vi "Add Dummy Grand Children.vi"(8 "error in (no error)":errorcluster, 9 "Folder Names":string[](array[string]), 10 "Parent Tag":string, 11 "Tree In":refnum<vi>) -> (0 "error out":errorcluster, 1 "Folder Names Dup":string[](array[string]), 2 "Parent Tag Dup":string, 3 "Tree Out":refnum<vi>)   [LabVIEW 2018, in "Tree Browser.lvlib"]
doc: "Adds a placeholder grandchild under each child of the parent node where the child directory listing contains folders. This means the tree can display the expand/contract symbol.\n\nNote that all the grandchildren aren't added to the tree here (ie. the full directory listing of a child) because it is simply too slow to build the tree this way (for example navigating to C:\\Windows which is roughly 20k nested folders will make LabVIEW crawl)."
uses:
  Tree Browser.lvlib
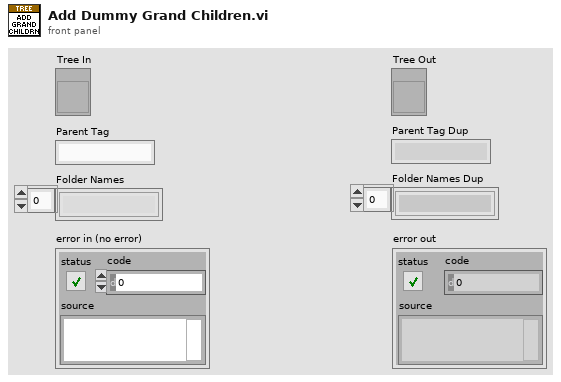
[diagram p1: front panel]
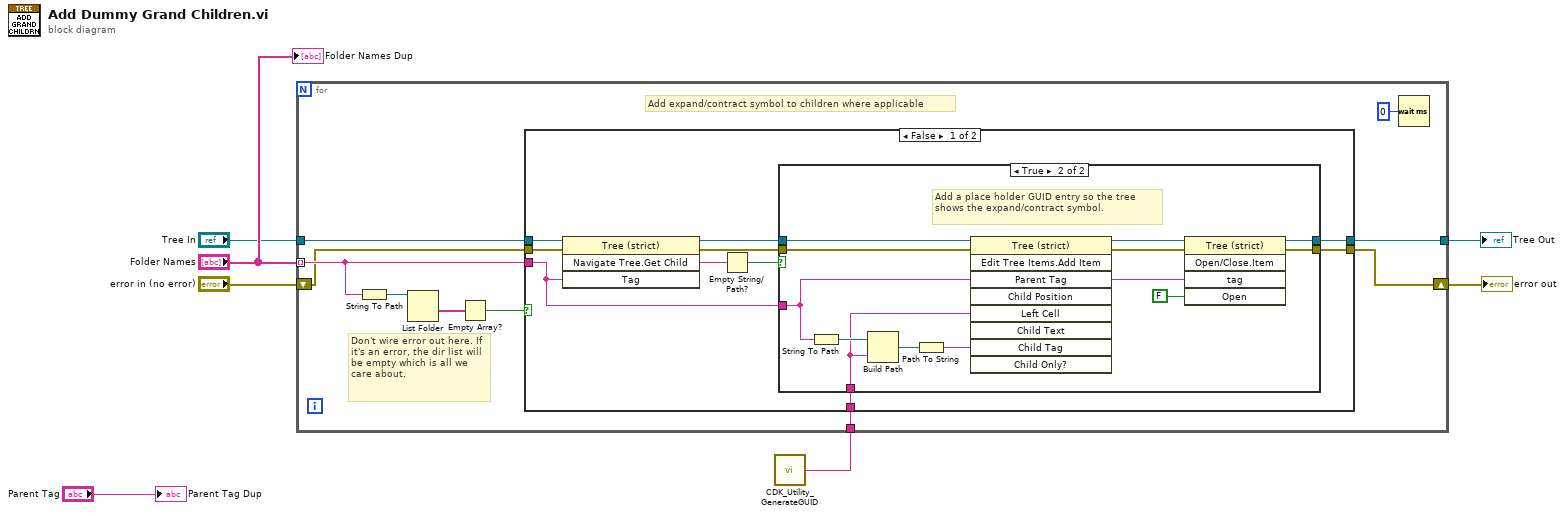
[diagram p0: block diagram]
diagram:
  n1 = call <resource>:"CDK_Utility_GenerateGUID.vi"() -> ("GUID"=w1:string)  [unwired: 9 in]
  n2 = for {
    tunnel: "Tree In" -> [w16]
    tunnel: "Folder Names" -> [w15] mode=indexing
    tunnel: w1 -> [w14]
    tunnel: [w13] -> w4
    shift-right: [w11] -> w2
    shift-left: "error in (no error)" -> [w12]
    # "Don't wire error out here. If it's an error, the dir list will be empty which is all we care about."
    # "Add expand/contract symbol to children where applicable"
    n3 = String To Path(string=w15) -> (path=w9:path)
    n4 = List Folder(path=w9) -> (folder names=w10:string[])  [unwired: 3 in, 3 out]
    n5 = Empty Array?(array=w10) -> (empty?=w17:bool)
    n6 = case shown="False" w17 {
      tunnel: w16 -> [w26 w43]
      tunnel: w15 -> [w23 _]
      tunnel: w14 -> [w22 _]
      tunnel: [w21 w43] -> w13
      tunnel: w12 -> [w20 w42]
      tunnel: [w18 w42] -> w11
      frame False {
        n7 = invoke class="Tree (strict)" method="Navigate Tree.Get Child"(reference=w26, error in=w20, "Tag"=w23) -> (reference out=w24:refnum<vi>, error out=w19:errorcluster, "Navigate Tree:Get Child"=w27:string)  [unwired: 1 in, 1 out]
        n8 = Empty String/Path?(string/path=w27) -> (empty?=w25:bool)
        n9 = case shown="True" w25 {
          tunnel: w24 -> [w29 w41]
          tunnel: w23 -> [_ w33]
          tunnel: w22 -> [_ w37]
          tunnel: [w29 w34] -> w21
          tunnel: w19 -> [w28 w32]
          tunnel: [w28 w30] -> w18
          frame False {
            # "The node already has children."
          }
          frame True {
            # "Add a place holder GUID entry so the tree shows the expand/contract symbol."
            n10 = String To Path(string=w33) -> (path=w40:path)
            n11 = Build Path(base path=w40, name or relative path=w37) -> (appended path=w39:path)
            n12 = Path To String(path=w39) -> (string=w38:string)
            n13 = invoke class="Tree (strict)" method="Edit Tree Items.Add Item"(reference=w41, error in=w32, "Parent Tag"=w33, "Left Cell"=w37, "Child Tag"=w38) -> (reference out=w36:refnum<vi>, error out=w31:errorcluster)  [unwired: 4 in, 7 out]
            n14 = invoke class="Tree (strict)" method="Open/Close.Item"(reference=w36, error in=w31, "tag"=w33, "Open"=FALSE ("Open?")) -> (reference out=w34:refnum<vi>, error out=w30:errorcluster)  [unwired: 1 in, 3 out]
          }
        }
      }
      frame True {
      }
    }
    n15 = Wait (ms)(milliseconds to wait=u32 0) -> ()  [unwired: 1 out]
  }
  "Tree Out" <- w4
  "error out" <- w2
  "Parent Tag Dup" <- "Parent Tag"
  "Folder Names Dup" <- "Folder Names"
